vi "CamUpdateSelectorRect.vi"(9 "large cam ref":refnum<vi>, 10 "XVerticalSlide":refnum<vi>, 11 "XHorizontalSlide":refnum<vi>) -> ()   [LabVIEW 2019]
uses:
  controls/xHorizontalSlide/XHorizontalSlide.xctl
  controls/xVerticalSlide/XVerticalSlide.xctl
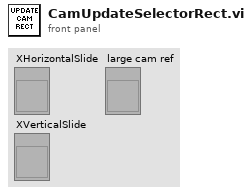
[diagram p1: front panel]
types:
  T1 = cluster{"Width":i16, "Style":enum32{"Solid", "Dash", "Dot", "DashDot", "DashDotDot"}}
  T2 = cluster{"left":i16, "top":i16, "right":i16, "bottom":i16}
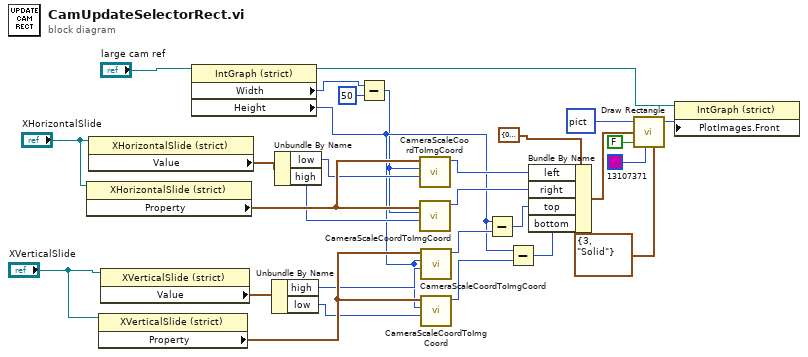
[diagram p0: block diagram]
diagram:
  n1 = property class="XHorizontalSlide (strict)"(reference="XHorizontalSlide") -> ("Property"=w19:cluster{"min":i16, "max":i16})  [unwired: 1 in, 2 out]
  n2 = property class="XHorizontalSlide (strict)"(reference="XHorizontalSlide") -> ("Value"=w15:cluster{"low":i16, "high":i16})  [unwired: 1 in, 2 out]
  n3 = property class="XVerticalSlide (strict)"(reference="XVerticalSlide") -> ("Property"=w18:cluster{"min":i16, "max":i16})  [unwired: 1 in, 2 out]
  n4 = property class="XVerticalSlide (strict)"(reference="XVerticalSlide") -> ("Value"=w14:cluster{"low":i16, "high":i16})  [unwired: 1 in, 2 out]
  n5 = property class="IntGraph (strict)"(reference="large cam ref") -> (reference out=w16:refnum<vi>, "Width"=w2:u32, "Height"=w4:u32)  [unwired: 1 in, 1 out]
  n6 = Unbundle By Name(w14) -> ("high"=w11:i16, "low"=w10:i16)
  n7 = Unbundle By Name(w15) -> ("low"=w13:i16, "high"=w12:i16)
  n8 = Subtract(x=w2, y=u32 50) -> (x-y=w1:u32)
  n9 = call "CameraScaleCoordToImgCoord.vi"("value"=w13, "img size"=w1, "scale bounds"=w19) -> ("coord out"=w23:i32)  [unwired: 8 in]
  n10 = call "CameraScaleCoordToImgCoord.vi"("value"=w12, "img size"=w1, "scale bounds"=w19) -> ("coord out"=w22:i32)  [unwired: 8 in]
  n11 = call "CameraScaleCoordToImgCoord.vi"("value"=w11, "img size"=w4, "scale bounds"=w18) -> ("coord out"=w7:i32)  [unwired: 8 in]
  n12 = call "CameraScaleCoordToImgCoord.vi"("value"=w10, "img size"=w4, "scale bounds"=w18) -> ("coord out"=w6:i32)  [unwired: 8 in]
  n13 = Subtract(x=w4, y=w7) -> (x-y=w5:u32)
  n14 = Subtract(x=w4, y=w6) -> (x-y=w8:u32)
  n15 = Bundle By Name(cluster=T2 {"left"=0, "top"=0, "right"=0, "bottom"=0} ("rect"), "left"=w23, "right"=w22, "top"=w5, "bottom"=w8) -> (w26:T2)
  n16 = call <vilib>:"Draw Rectangle.vi"("picture"=picture data[5B], "rect"=w26, "fill?(F)"=FALSE, "color(black)"=u32 13107371, "pen"=T1 {"Width"=3, "Style"=enum."Solid"}) -> ("new picture"=w24:picture)  [unwired: 4 in]
  n17 = property class="IntGraph (strict)"(reference=w16, "PlotImages.Front"=w24) -> ()  [unwired: 1 in, 2 out]
